vi "initialize.vi"(0 "HGF_ImaqDx":refnum<class "HGF_ImaqDx.lvclass">, 3 "initializationData":variant, 5 "error in (no error)":errorcluster, 7 "binaryString":string, 8 "I8 Array":i8[](array[numeric]), 9 "prependSize? (T)":bool, 11 "byteOrder (0:big-endian, network order)":T1(ring)) -> (14 "dup HGF_ImaqDx":refnum<class "HGF_ImaqDx.lvclass">, 17 "found?":bool, 19 "error out":errorcluster)   [LabVIEW 2014, in "HGF_IMAQ.lvlib" / "HGF_ImaqDx.lvclass"]
doc: "This is a dynamic dispatch VI to be implemented by child classes to initialize their attributes.\n\n<B>Recommendation:</B> Use Variant for initialization data."
uses:
  HGF_ImaqDx.lvclass
  HGF_IMAQDevice/HGF_IMAQDevice.lvclass
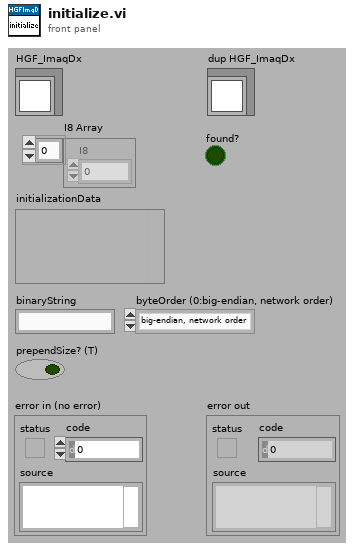
[diagram p1: front panel]
types:
  T1 = enum16{"big-endian, network order", "native, host order", "little-endian"}
  T2 = typedef "HGF_IMAQ.lvlib/HGF_IMAQDevice.lvclass/Control Mode.ctl" = enum16{"Controller", "Listener"}
  T3 = typedef "IMAQdx.ctl" = refnum<k21>
  T4 = cluster{"Video Mode":u32, "Video Mode Name":string}[]
  T5 = typedef "NI_Vision_Acquisition_Software.lvlib/IMAQdx Attribute Type.ctl" = enum32{"U32", "I64", "DBL", "String", "Enum", "Bool", "Command"}
  T6 = cluster{"Attribute Type":T5, "Readable":bool, "Writable":bool, "Attribute Name":string}[]
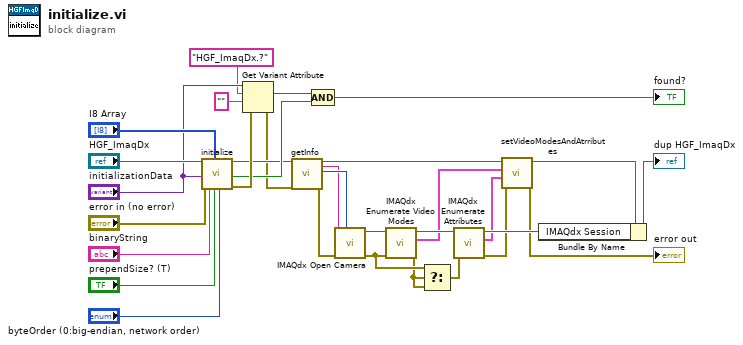
[diagram p0: block diagram]
diagram:
  n1 = call-parent "initialize.vi"("HGF_IMAQDevice"="HGF_ImaqDx", "initializationData"="initializationData", "error in (no error)"="error in (no error)", "binaryString"="binaryString", "I8 Array"="I8 Array", "prependSize? (T)"="prependSize? (T)", "byteOrder (0:big-endian, network order)"="byteOrder (0:big-endian, network order)") -> ("dup HGF_IMAQDevice"=w17:refnum<class "HGF_ImaqDx.lvclass">, "found?"=w22:bool, "error out"=w24:errorcluster)  [unwired: 10 out]
  n2 = Get Variant Attribute(Variant="initializationData", name="HGF_ImaqDx.?", default value (empty Variant)="", error in=w24) -> (found=w23:bool, error out=w16:errorcluster)  [unwired: 2 out]
  n3 = call "getInfo.vi"("HGF_IMAQDevice"=w17, "error in (no error)"=w16) -> ("dup HGF_IMAQDevice"=w9:refnum<class "HGF_ImaqDx.lvclass">, "cameraName"=w13:string, "controlMode"=w15:T2, "error out"=w14:errorcluster)  [unwired: 12 in, 2 out]
  n4 = Compound Arithmetic op=AND(w23, w22) -> (→"found?":bool)
  n5 = call <vilib>:"IMAQdx Open Camera.vi"("Camera Control Mode"=w15, "error in"=w14, "Session In"=w13) -> ("error out"=w3:errorcluster, "Session Out"=w11:T3)  [unwired: 7 out]
  n6 = call <vilib>:"IMAQdx Enumerate Video Modes.vi"("error in"=w3, "Session In"=w11) -> ("error out"=w2:errorcluster, "Video Modes"=w7:T4, "Session Out"=w12:T3)  [unwired: 6 in, 1 out]
  n7 = Select(t=w3, s=w2, f=w2) -> (s? t:f=w1:errorcluster)
  n8 = call <vilib>:"IMAQdx Enumerate Attributes.vi"("error in"=w1, "Session In"=w12) -> ("error out"=w5:errorcluster, "Attribute Information Array"=w6:T6, "Session Out"=w10:T3)  [unwired: 7 in]
  n9 = call "setVideoModesAndAtrributes.vi"("error in (no error)"=w5, "Attribute Information"=w6, "Video Modes"=w7, "HGF_IMAQDevice in"=w9) -> ("error out"=→"error out":errorcluster, "HGF_IMAQDevice out"=w8:refnum<class "HGF_ImaqDx.lvclass">)  [unwired: 6 in]
  n10 = Bundle By Name(cluster=w8, "IMAQdx Session"=w10) -> (→"dup HGF_ImaqDx":refnum<class "HGF_ImaqDx.lvclass">)
